vi "Update Traffic Light.vi"(6 "Color state in":T2[](array[typedef]), 7 "Time in":i32[](array[numeric]), 8 "Color times":T1, 9 "Blinking":bool, 10 "Sync in":bool) -> (2 "Sync out":bool, 4 "Color state out":T2[](array[typedef]), 5 "Time out":i32[](array[numeric]))   [LabVIEW 2018]
uses:
  Color states.ctl
  Color times.ctl
panel:
  out "index":i32
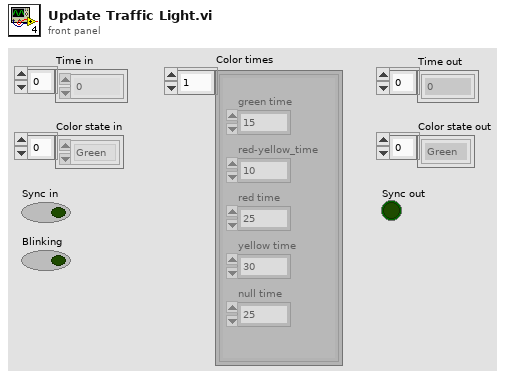
[diagram p1: front panel]
types:
  T1 = typedef "Color times.ctl" = cluster{"yellow time":i32, "red-yellow_time":i32, "green time":i32, "red time":i32, "null time":i32}[]
  T2 = typedef "Color states.ctl" = enum16{"Green", "Red-Yellow", "Yellow", "Red", "Null"}
  T3 = cluster{"yellow time":i32, "red-yellow_time":i32, "green time":i32, "red time":i32, "null time":i32}
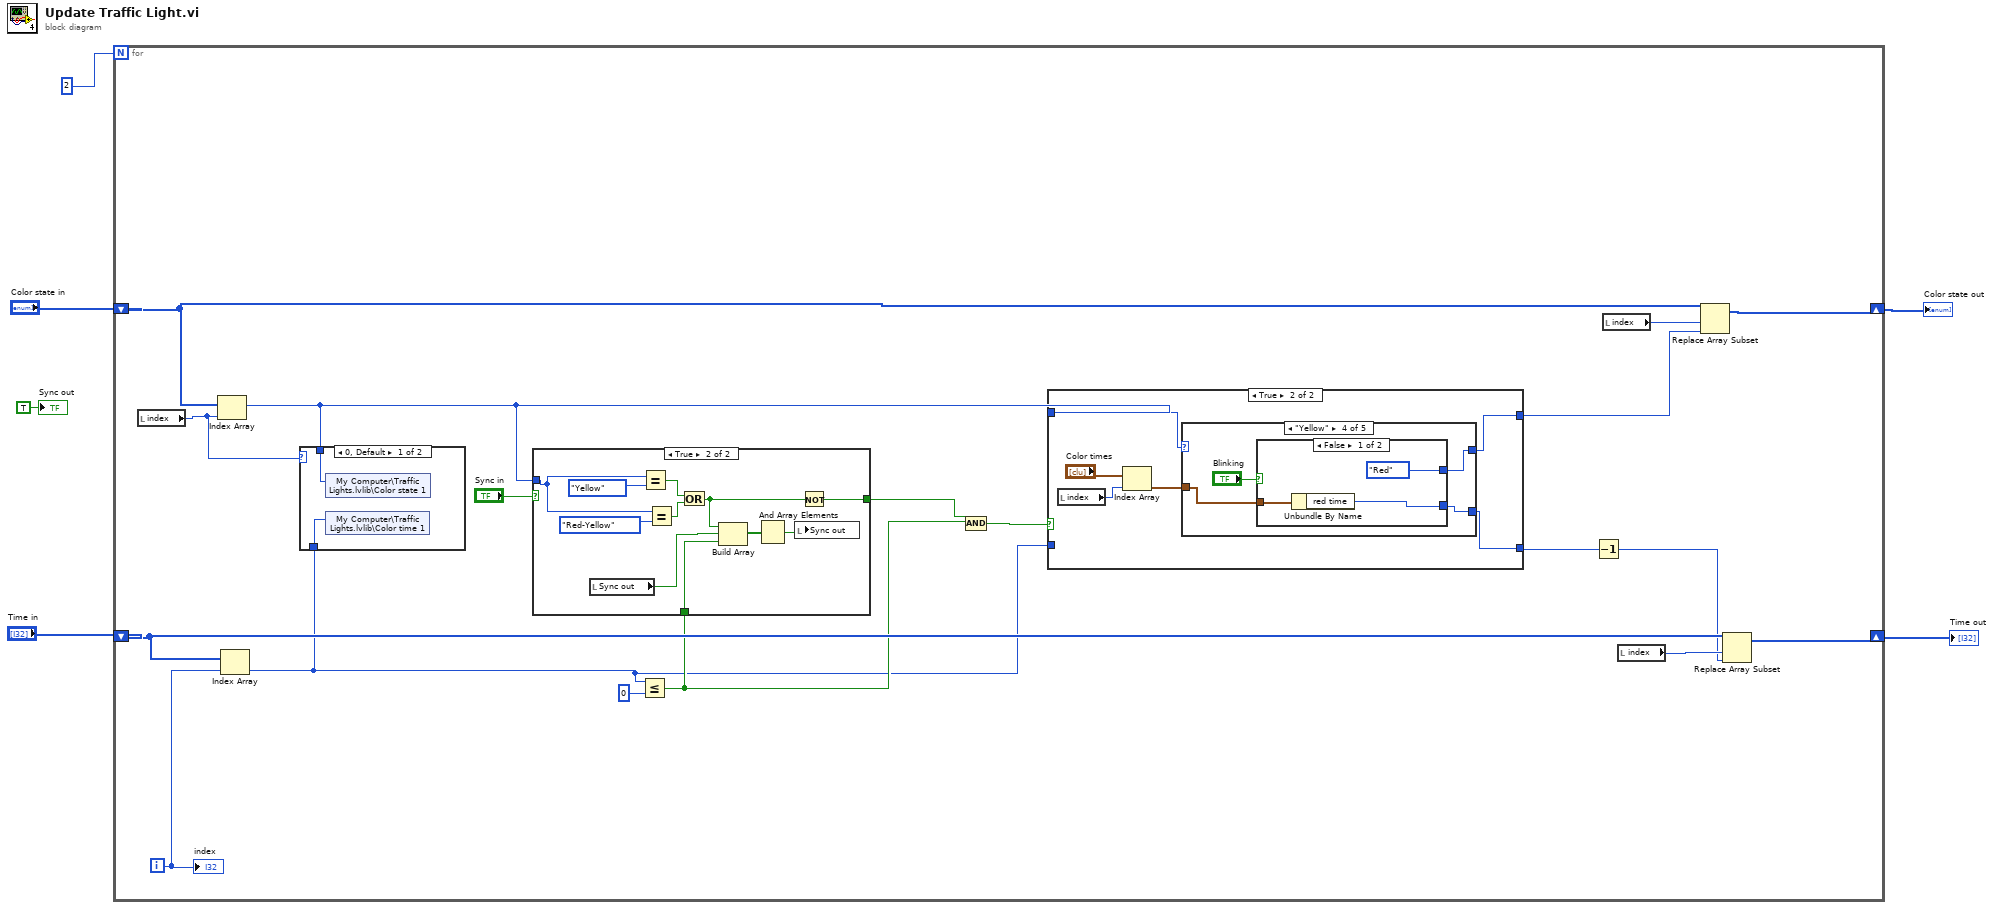
[diagram p0: block diagram]
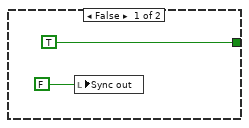
[diagram p2: hidden frame]
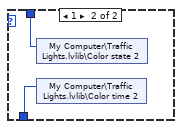
[diagram p3: hidden frame]
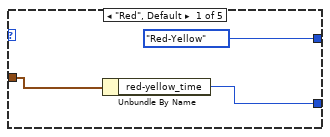
[diagram p5: hidden frame]
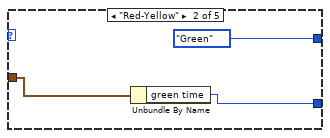
[diagram p6: hidden frame]
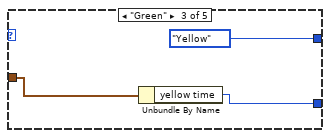
[diagram p7: hidden frame]
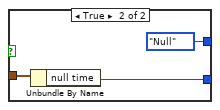
[diagram p8: hidden frame]
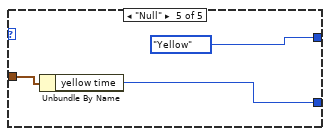
[diagram p9: hidden frame]
diagram:
  n1 = for {
    N: 2 -> [_]
    shift-right: [w22] -> w4
    shift-left: "Color state in" -> [w23]
    shift-right: [w20] -> w2
    shift-left: "Time in" -> [w21]
    i -> [w19]
    n2 = local read "index"() -> (w16:i32)
    n3 = Index Array "Index Array"(array=w23, index=w16) -> (element=w13:T2)
    n4 = Index Array "Index Array"(array=w21, index=w19) -> (element=w10:i32)
    n5 = case shown="0, Default" w16 {
      tunnel: w10 -> [w39 w41]
      tunnel: w13 -> [w38 w40]
      frame 0, Default {
        n6 = shared-variable "My Computer\\Traffic Lights.lvlib\\Color state 1"(w38) -> ()  [unwired: 1 in, 1 out]
        n7 = shared-variable "My Computer\\Traffic Lights.lvlib\\Color time 1"(w39) -> ()  [unwired: 1 in, 1 out]
      }
      frame 1 {
        n8 = shared-variable "My Computer\\Traffic Lights.lvlib\\Color state 2"(w40) -> ()  [unwired: 1 in, 1 out]
        n9 = shared-variable "My Computer\\Traffic Lights.lvlib\\Color time 2"(w41) -> ()  [unwired: 1 in, 1 out]
      }
    }
    n10 = Less Or Equal?(x=w10, y=0) -> (x <= y?=w11:bool)
    n11 = case shown="True" "Sync in" {
      tunnel: [TRUE w32] -> w14
      tunnel: w13 -> [_ w36]
      tunnel: w11 -> [_ w29]
      frame False {
        n12 = local write "Sync out"(FALSE ("Sync out")) -> ()
      }
      frame True {
        n13 = local read "Sync out"() -> (w28:bool)
        n14 = Equal?(x=w36, y=Color_states."Yellow") -> (x = y?=w33:bool)
        n15 = Equal?(x=w36, y=Color_states."Red-Yellow") -> (x = y?=w34:bool)
        n16 = Or(x=w33, y=w34) -> (x .or. y?=w27:bool)
        n17 = Build Array(w27, w28, w29) -> (w30:bool[])
        n18 = And Array Elements(Boolean array=w30) -> (logical AND=w31:bool)
        n19 = local write "Sync out"(w31) -> ()
        n20 = Not(x=w27) -> (.not. x?=w32:bool)
      }
    }
    n21 = And(x=w14, y=w11) -> (x .and. y?=w15:bool)
    n22 = case shown="True" w15 {
      tunnel: w13 -> [w43 w47]
      tunnel: [w43 w49] -> w24
      tunnel: [w42 w48] -> w8
      tunnel: w10 -> [w42 _]
      frame False {
      }
      frame True {
        n23 = local read "index"() -> (w44:i32)
        n24 = Index Array(array="Color times", index=w44) -> (element=w45:T3)
        n25 = case shown="\"Yellow\"" w47 {
          tunnel: [Color_states."Red-Yellow" Color_states."Green" Color_states."Yellow" w62 Color_states."Yellow"] -> w49
          tunnel: [w51 w53 w56 w59 w70] -> w48
          tunnel: w45 -> [w50 w54 w57 w60 w69]
          frame "Red", Default {
            n26 = Unbundle By Name(w50) -> ("red-yellow_time"=w51:i32)
          }
          frame "Red-Yellow" {
            n27 = Unbundle By Name(w54) -> ("green time"=w53:i32)
          }
          frame "Green" {
            n28 = Unbundle By Name(w57) -> ("yellow time"=w56:i32)
          }
          frame "Yellow" {
            n29 = case shown="False" "Blinking" {
              tunnel: [w64 w67] -> w59
              tunnel: [Color_states."Red" Color_states."Null"] -> w62
              tunnel: w60 -> [w63 w66]
              frame False {
                n30 = Unbundle By Name(w63) -> ("red time"=w64:i32)
              }
              frame True {
                n31 = Unbundle By Name(w66) -> ("null time"=w67:i32)
              }
            }
          }
          frame "Null" {
            n32 = Unbundle By Name(w69) -> ("yellow time"=w70:i32)
          }
        }
      }
    }
    n33 = Decrement(x=w8) -> (x-1=w7:i32)
    n34 = local read "index"() -> (w18:i32)
    n35 = local read "index"() -> (w17:i32)
    n36 = Replace Array Subset "Replace Array Subset"(array=w23, new element=w24, index=w18) -> (w22:T2[])
    n37 = Replace Array Subset "Replace Array Subset"(array=w21, new element=w7, index=w17) -> (w20:i32[])
    "index" <- w19
  }
  "Time out" <- w2
  "Color state out" <- w4
  "Sync out" <- TRUE ("Sync out")
